vi "Logout.vi"(4 "Source (\"\")":string, 8 "error in (no error)":errorcluster, 11 "VISA resource name":refnum<visa-resource-name>) -> (0 "error out":errorcluster, 3 "VISA resource name out":refnum<visa-resource-name>)   [LabVIEW 2020, in "Yokogawa GX Series.lvlib"]
doc: "This VI logouts from the instrument. Then it can not re-login."
uses:
  <instrlib>/Yokogawa GX Series/Yokogawa GX Series.lvlib
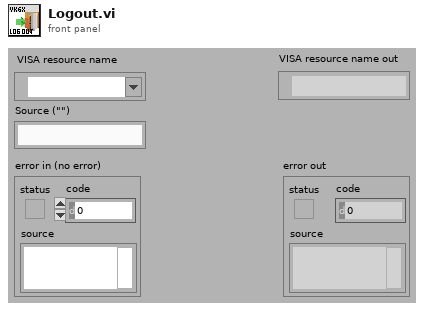
[diagram p1: front panel]
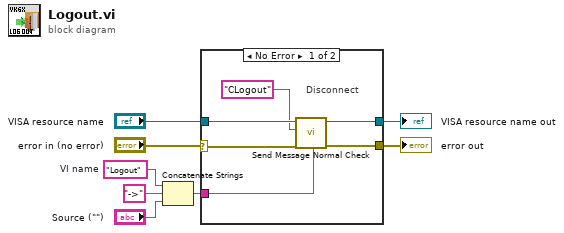
[diagram p0: block diagram]
diagram:
  w8 = "Logout"  # VI name
  n1 = Concatenate Strings(w8, "->", "Source (\"\")") -> (w4:string)
  n2 = case shown="No Error" "error in (no error)" {
    selector: "error in (no error)" -> [w9 w15]
    tunnel: "VISA resource name" -> [w14 w16]
    tunnel: w4 -> [w12 _]
    tunnel: [w11 w16] -> w3
    tunnel: [w10 w15] -> w2
    frame No Error {
      # "Disconnect"
      n3 = call <instrlib>:"Send Message Normal Check.vi"("Source (\"\")"=w12, "error in (no error)"=w9, "Send Message (\"\")"="CLogout", "VISA resource name"=w14) -> ("error out"=w10:errorcluster, "VISA resource name out"=w11:refnum<visa-resource-name>)  [unwired: 2 in, 4 out]
    }
    frame Error {
    }
  }
  "error out" <- w2
  "VISA resource name out" <- w3
